vi "HIOKI PW3390 OPC.vi"(8 "error in (no error)":errorcluster, 11 "VISA Resource":refnum<visa-resource-name>) -> (0 "error out":errorcluster, 2 "OPC":u8, 3 "VISA Resource out":refnum<visa-resource-name>)   [LabVIEW 2009]
doc: "outputs 1 after processing the commands before the \"HIOKI PW3390 OPC.vi\"."
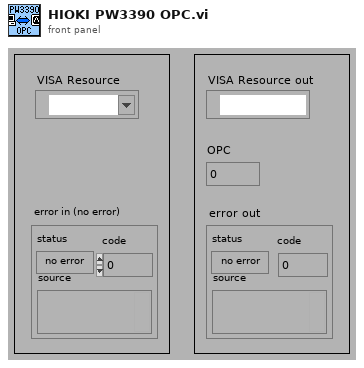
[diagram p1: front panel]
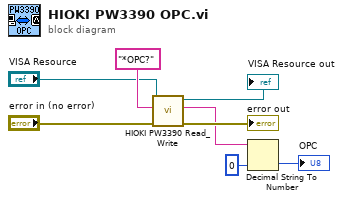
[diagram p0: block diagram]
diagram:
  n1 = call <instrlib>:"HIOKI PW3390 Read_Write.vi"("error in (no error)"="error in (no error)", "data in"="*OPC?", "VISA Resource"="VISA Resource") -> ("error out"=→"error out":errorcluster, "data out"=w5:string, "VISA Resource out"=→"VISA Resource out":refnum<visa-resource-name>)  [unwired: 6 in]
  n2 = Decimal String To Number(string=w5, default (0L)=u8 0 ("デフォルト (0L)")) -> (number=→"OPC":u8)  [unwired: 1 in, 1 out]
